vi "Read Second Level VR.vi"(5 "Tag":string, 7 "Section":string, 8 "error in (no error)":errorcluster, 11 "Variant Repository In":variant) -> (0 "error out":errorcluster, 2 "Value":string, 3 "Variant Repository Out":variant)   [LabVIEW 2017, in "Front Panel Publisher.lvlib"]
uses:
  Front Panel Publisher.lvlib
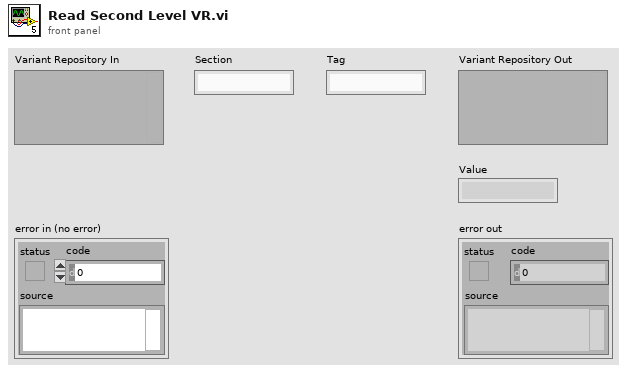
[diagram p1: front panel]
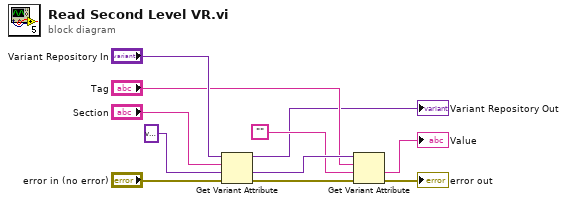
[diagram p0: block diagram]
diagram:
  n1 = Get Variant Attribute(Variant="Variant Repository In", name="Section", default value (empty Variant)=variant, error in="error in (no error)") -> (duplicate Variant=→"Variant Repository Out":variant, value=w8:variant, error out=w5:errorcluster)  [unwired: 1 out]
  n2 = Get Variant Attribute(Variant=w8, name="Tag", default value (empty Variant)="", error in=w5) -> (value=→"Value":string, error out=→"error out":errorcluster)  [unwired: 2 out]
